vi "ex6.vi"() -> ()   [LabVIEW 2022 SP3]
panel:
  out "Execution Time [ms]":u32
  in  "Loop Delay [ms]":dbl
  out "Num 2":dbl
  out "Num 1":dbl
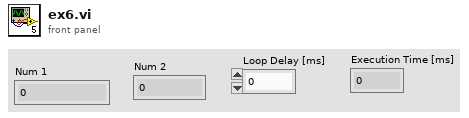
[diagram p1: front panel]
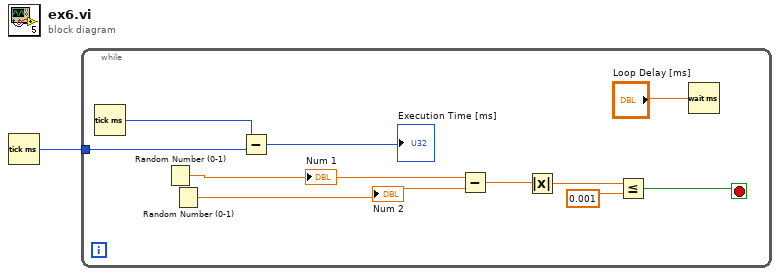
[diagram p0: block diagram]
diagram:
  n1 = Tick Count (ms)() -> (millisecond timer value=w1:u32)
  n2 = while {
    tunnel: w1 -> [w3]
    stop <- w8 stop-if-true
    n3 = Tick Count (ms)() -> (millisecond timer value=w4:u32)
    n4 = Random Number (0-1)() -> (number: 0 to 1=w7:dbl)
    "Num 1" <- w7
    n5 = Random Number (0-1)() -> (number: 0 to 1=w6:dbl)
    "Num 2" <- w6
    n6 = Subtract(x=w4, y=w3) -> (x-y=→"Execution Time [ms]":u32)
    n7 = Subtract(x=w7, y=w6) -> (x-y=w11:dbl)
    n8 = Absolute Value(x=w11) -> (abs(x)=w10:dbl)
    n9 = Less Or Equal?(x=w10, y=0.001) -> (x <= y?=w8:bool)
    n10 = Wait (ms)(milliseconds to wait="Loop Delay [ms]") -> ()  [unwired: 1 out]
  }
